vi "Get Active Line Tag Name.vi"(8 "error in (no error)":errorcluster, 11 "Pairing Tab Refs":T1) -> (0 "error out":errorcluster, 2 "Tag Name":string)   [LabVIEW 2015, in "E2E Tag Exchange editor node.lvclass"]
uses:
  E2E Tag Exchange editor node.lvclass
  Tag Exchange Tab References.ctl
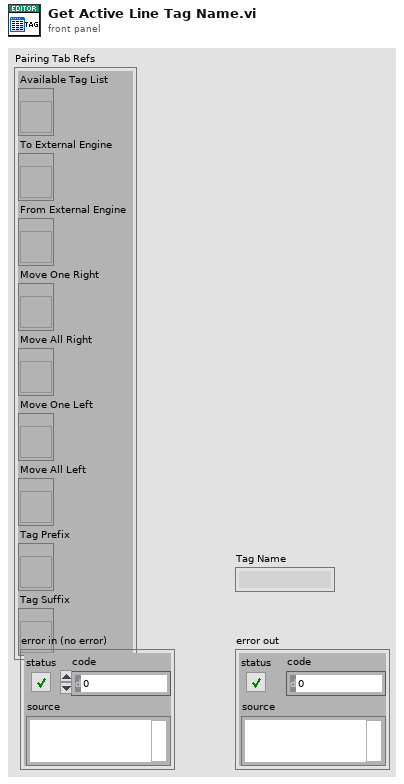
[diagram p1: front panel]
types:
  T1 = typedef "E2E Tag Exchange editor node.lvclass/Tag Exchange Tab References.ctl" = cluster{"Available Tag List":refnum<vi>, "To External Engine":refnum<vi>, "From External Engine":refnum<vi>, "Move One Right":refnum<vi>, "Move All Right":refnum<vi>, "Move One Left":refnum<vi>, "Move All Left":refnum<vi>, "Tag Prefix":refnum<vi>, "Tag Suffix":refnum<vi>}
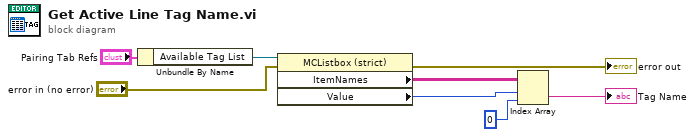
[diagram p0: block diagram]
diagram:
  n1 = Unbundle By Name("Pairing Tab Refs") -> ("Available Tag List"=w7:refnum<vi>)
  n2 = property class="MCListbox (strict)"(reference=w7, error in="error in (no error)") -> (error out=→"error out":errorcluster, "ItemNames"=w6:string[][], "Value"=w5:i32)  [unwired: 1 out]
  n3 = Index Array(array=w6, index (row)=w5, index (col)=0 ("disabled index (col)")) -> (element=→"Tag Name":string)
